vi "Table_SortArrayFromHightoLow.vi"(11 "Channels":i32[](array[numeric])) -> (3 "Array":i32[](array[numeric]))   [LabVIEW 2012, in "TableSupportLib.lvlib"]
uses:
  TableSupportLib.lvlib
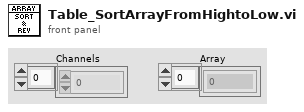
[diagram p1: front panel]
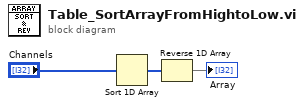
[diagram p0: block diagram]
diagram:
  n1 = Sort 1D Array(array="Channels") -> (sorted array=w2:i32[])
  n2 = Reverse 1D Array(array=w2) -> (reversed array=→"Array":i32[])
